vi "Execute.vi"(8 "error in (no error)":errorcluster, 10 "Abstract Producer in":refnum<class "Abstract Producer.lvclass">, 11 "Count Response Message in":refnum<class "Count Response Message.lvclass">) -> (0 "error out":errorcluster, 2 "Abstract Producer out":refnum<class "Abstract Producer.lvclass">, 3 "Count Response Message out":refnum<class "Count Response Message.lvclass">)   [LabVIEW 2017, in "Count Response Message.lvclass"]
uses:
  Count Response Message.lvclass
  Producer/Abstract Producer/Abstract Producer.lvclass
  Message List Action.ctl
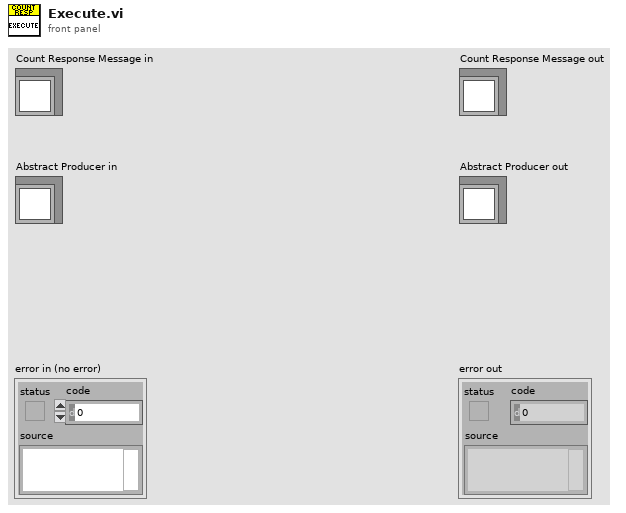
[diagram p1: front panel]
types:
  T1 = typedef "Message List Action.ctl" = enum16{"Get", "Add", "Reset"}
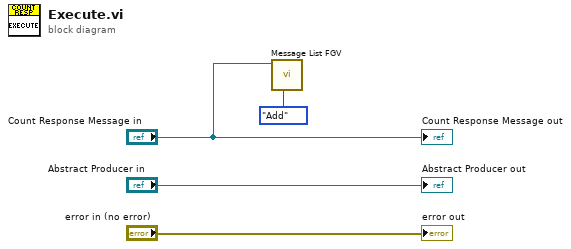
[diagram p0: block diagram]
diagram:
  n1 = call "Message List FGV.vi"("Action (Get)"=Message_List_Action."Add", "Message Object"="Count Response Message in") -> ()  [unwired: 8 in, 2 out]
  "error out" <- "error in (no error)"
  "Count Response Message out" <- "Count Response Message in"
  "Abstract Producer out" <- "Abstract Producer in"
